vi "SubTest_SelectData.vi"(8 "error in (no error)":errorcluster) -> (0 "error out":errorcluster, 1 "Selected?T":bool)   [LabVIEW 2014, in "TableLogger_CSV_Actor.lvlib" / "TableLogger_CSV_Actor.lvclass"]
uses:
  TableLogger_CSV_Actor.lvclass
  TableLogger_Actor/TableLoggerConfig.ctl
  TableLogger_Actor/TableLoggerTypes.ctl
  TableLogger_Actor/TableLoggerBackupConfig.ctl
  TableLogger_Actor/SelectConditionCriteria.ctl
  TableLogger_SQLite_Actor/SelectConditions.ctl
  TableLogger_Actor/TableLogger_Actor.lvlib
panel:
  # "This example to check CSV update on Tablelogger"
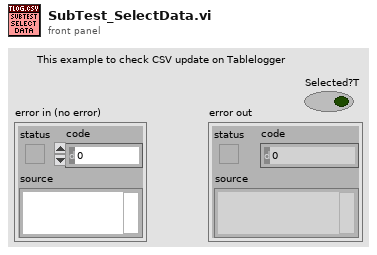
[diagram p1: front panel]
types:
  T1 = typedef "TableLogger_Actor.lvlib/SelectConditionCriteria.ctl" = cluster{"Condition Data":variant[], "Recent N.Rows":string, "Select Type":T2}
  T2 = typedef "TableLogger_Actor.lvlib/SelectConditions.ctl" = enum16{"Select All", "AND Operator", "Recent Rows", "OR Operator", "BETWEEN Operator"}
  T3 = cluster{"Numeric Data":i32, "Float Data":dbl, "String Data":string, "Enum Data":enum16{"Enum Item 1", "Enum Item 2"}, "Array Data 2":i32[], "Cluster 2":cluster{"String":string, "Array Data 2":i32[]}, "Cluster 3":cluster{"Cluster78":cluster{"Array Data 2":i32[]}}, "Enum Data 2":enum16{"Enum Item 1", "Enum Item 2"}, "String Data 2":string, "Float Data 2":dbl, "Array Data":i32[], "Array A":cluster{"String A":string, "Array B":cluster{"String B":string, "Array B 2":cluster{"String B":string}[]}[], "Array B 2":cluster{"String B":string}[]}[]}[]
  T4 = typedef "TableLogger_Actor.lvlib/TableLoggerConfig.ctl" = cluster{"TableLogger":T5, "DB File Path":path, "DB Backup Config":T6}
  T5 = typedef "TableLogger_Actor.lvlib/TableLoggerTypes.ctl" = enum16{"CSV Logger", "SQLite Logger"}
  T6 = typedef "TableLogger_Actor.lvlib/TableLoggerBackupConfig.ctl" = cluster{"Directory":path, "UTC Time Format":bool, "On Launch":bool, "Interval (Hours)":dbl, "Size Multiples (Bytes)":i32}
  T7 = cluster{"Numeric Data":i32, "Float Data":dbl, "String Data":string, "Enum Data":enum16{"Enum Item 1", "Enum Item 2"}}
  T8 = cluster{"Test Start Timestamp":timestamp, "Test End Timestamp":timestamp, "Test Jig Location":string, "Location Time Offset":string, "Test Jig ID":string, "Test Jig Fluid":enum16{"Liquid", "Gas"}, "Test Jig Flow":enum16{"Low", "High"}, "Control Board SN":string, "Site Number":i32, "Operator ID":string, "Operation Number":string, "DUT Serial Number":string, "DUT Product Number":string, "DUT Flow Range":i32, "DUT FW Revision":string, "DUT TP1 Offset":dbl, "DUT TP2 Offset":dbl, "DUT Cut Off1":dbl, "DUT Cut Off2":dbl, "PreCal Flow Meas":cluster{"FC Flow Set":dbl, "FM Flow Measure":dbl, "UUT Data":dbl}[], "PostCal Flow Meas":cluster{"FC Flow Set":dbl, "FM Flow Measure":dbl, "UUT Data":dbl}[], "DUT_Coeff":dbl[], "DUT_Flow_Error":dbl[], "Calibration Result":enum16{"Pass", "Fail"}}
  T9 = cluster{"Numeric Data":i32, "Float Data":dbl, "String Data":string, "Enum Data":enum16{"Enum Item 1", "Enum Item 2"}, "Array Data 2":i32[], "Cluster 2":cluster{"String":string, "Array Data 2":i32[]}, "Cluster 3":cluster{"Cluster78":cluster{"Array Data 2":i32[]}}, "Enum Data 2":enum16{"Enum Item 1", "Enum Item 2"}, "String Data 2":string, "Float Data 2":dbl, "Array Data":i32[], "Array A":cluster{"String A":string, "Array B":cluster{"String B":string, "Array B 2":cluster{"String B":string}[]}[], "Array B 2":cluster{"String B":string}[]}[]}
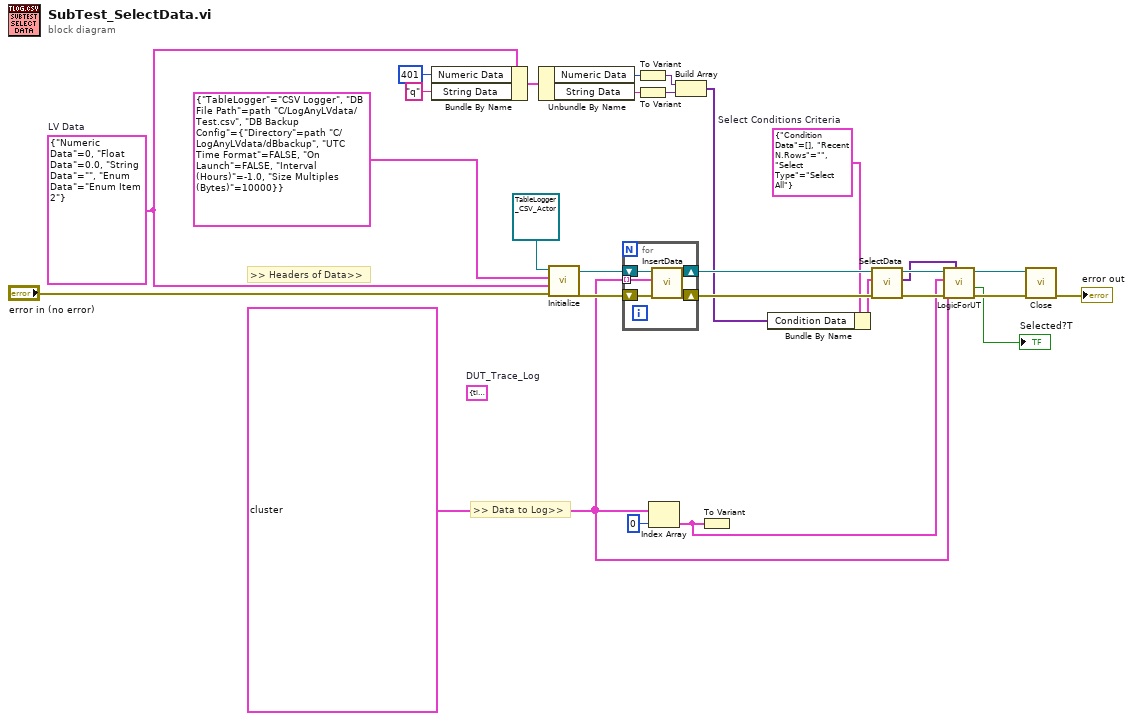
[diagram p0: block diagram]
diagram:
  w3 = T1 {"Condition Data"=[], "Recent N.Rows"="", "Select Type"=enum."Select All"}  # Select Conditions Criteria
  w15 = T3 [{"Numeric Data"=0, "Float Data"=0.0, "String Data"="", "Enum Data"=enum."Enum Item 1", "Array Data 2"=[0, 0, 0], "Cluster 2"={"String"="", "Array Data 2"=[0, 0, 0]}, "Cluster 3"={"Cluster78"={"Array Data 2"=[0, 0, 0]}}, "Enum Data 2"=enum."Enum Item 1", "String Data 2"="", "Float Data 2"=0.0, "Array Data"=[0, 0, 0, 4], "Array A"=[{"String A"="hello", "Array B"=[{"String B"="uq", "Array B 2"=[{"String B"="u"}, {"String B"="c"}, {"String B"="hello"}]}, {"String B"="c", "Array B 2"=[{"String B"="u"}, {"String B"="c"}, {"String B"="hello"}]}, {"String B"="hello", "Array B 2"=[{"String B"="u"}, {"String B"="c"}, {"String B"="hello"}]}], "Array B 2"=[{"String B"="u"}, {"String B"="c"}, {"String B"="hello"}]}, {"String A"="hello", "Array B"=[{"String B"="uP", "Array B 2"=[{"String B"="u"}, {"String B"="c"}, {"String B"="hello"}]}, {"String B"="c", "Array B 2"=[{"String B"="u"}, {"String B"="c"}, {"String B"="hello"}]}, {"String B"="hello", "Array B 2"=[{"String B"="u"}, {"String B"="c"}, {"String B"="hello"}]}], "Array B 2"=[{"String B"="u"}, {"String B"="c"}, {"String B"="hello"}]}]}, {"Numeric Data"=401, "Float Data"=0.0, "String Data"="q", "Enum Data"=enum."Enum Item 1", "Array Data 2"=[0, 0, 0], "Cluster 2"={"String"="", "Array Data 2"=[0, 0, 0]}, "Cluster 3"={"Cluster78"={"Array Data 2"=[0, 0, 0]}}, "Enum Data 2"=enum."Enum Item 1", "String Data 2"="", "Float Data 2"=0.0, "Array Data"=[0, 0, 0, 4], "Array A"=[{"String A"="hello", "Array B"=[{"String B"="uq", "Array B 2"=[{"String B"="u"}, {"String B"="c"}, {"String B"="hello"}]}, {"String B"="c", "Array B 2"=[{"String B"="u"}, {"String B"="c"}, {"String B"="hello"}]}, {"String B"="hello", "Array B 2"=[{"String B"="u"}, {"String B"="c"}, {"String B"="hello"}]}], "Array B 2"=[{"String B"="u"}, {"String B"="c"}, {"String B"="hello"}]}, {"String A"="hello", "Array B"=[{"String B"="uP", "Array B 2"=[{"String B"="u"}, {"String B"="c"}, {"String B"="hello"}]}, {"String B"="c", "Array B 2"=[{"String B"="u"}, {"String B"="c"}, {"String B"="hello"}]}, {"String B"="hello", "Array B 2"=[{"String B"="u"}, {"String B"="c"}, {"String B"="hello"}]}], "Array B 2"=[{"String B"="u"}, {"String B"="c"}, {"String B"="hello"}]}]}, {"Numeric Data"=0, "Float Data"=0.0, "String Data"="", "Enum Data"=enum."Enum Item 1", "Array Data 2"=[0, 0, 0], "Cluster 2"={"String"="", "Array Data 2"=[0, 0, 0]}, "Cluster 3"={"Cluster78"={"Array Data 2"=[0, 0, 0]}}, "Enum Data 2"=enum."Enum Item 1", "String Data 2"="", "Float Data 2"=0.0, "Array Data"=[0, 0, 0, 4], "Array A"=[{"String A"="hello", "Array B"=[{"String B"="uq", "Array B 2"=[{"String B"="u"}, {"String B"="c"}, {"String B"="hello"}]}, {"String B"="c", "Array B 2"=[{"String B"="u"}, {"String B"="c"}, {"String B"="hello"}]}, {"String B"="hello", "Array B 2"=[{"String B"="u"}, {"String B"="c"}, {"String B"="hello"}]}], "Array B 2"=[{"String B"="u"}, {"String B"="c"}, {"String B"="hello"}]}, {"String A"="hello", "Array B"=[{"String B"="uP", "Array B 2"=[{"String B"="u"}, {"String B"="c"}, {"String B"="hello"}]}, {"String B"="c", "Array B 2"=[{"String B"="u"}, {"String B"="c"}, {"String B"="hello"}]}, {"String B"="hello", "Array B 2"=[{"String B"="u"}, {"String B"="c"}, {"String B"="hello"}]}], "Array B 2"=[{"String B"="u"}, {"String B"="c"}, {"String B"="hello"}]}]}, {"Numeric Data"=0, "Float Data"=0.0, "String Data"="", "Enum Data"=enum."Enum Item 1", "Array Data 2"=[0, 0, 0], "Cluster 2"={"String"="", "Array Data 2"=[0, 0, 0]}, "Cluster 3"={"Cluster78"={"Array Data 2"=[0, 0, 0]}}, "Enum Data 2"=enum."Enum Item 1", "String Data 2"="", "Float Data 2"=0.0, "Array Data"=[0, 0, 0, 4], "Array A"=[{"String A"="hello", "Array B"=[{"String B"="uq", "Array B 2"=[{"String B"="u"}, {"String B"="c"}, {"String B"="hello"}]}, {"String B"="c", "Array B 2"=[{"String B"="u"}, {"String B"="c"}, {"String B"="hello"}]}, {"String B"="hello", "Array B 2"=[{"String B"="u"}, {"String B"="c"}, {"String B"="hello"}]}], "Array B 2"=[{"String B"="u"}, {"String B"="c"}, {"String B"="hello"}]}, {"String A"="hello", "Array B"=[{"String B"="uP", "Array B 2"=[{"String B"="u"}, {"String B"="c"}, {"String B"="hello"}]}, {"String B"="c", "Array B 2"=[{"String B"="u"}, {"String B"="c"}, {"String B"="hello"}]}, {"String B"="hello", "Array B 2"=[{"String B"="u"}, {"String B"="c"}, {"String B"="hello"}]}], "Array B 2"=[{"String B"="u"}, {"String B"="c"}, {"String B"="hello"}]}]}, {"Numeric Data"=0, "Float Data"=0.0, "String Data"="", "Enum Data"=enum."Enum Item 1", "Array Data 2"=[0, 0, 0], "Cluster 2"={"String"="", "Array Data 2"=[0, 0, 0]}, "Cluster 3"={"Cluster78"={"Array Data 2"=[0, 0, 0]}}, "Enum Data 2"=enum."Enum Item 1", "String Data 2"="", "Float Data 2"=0.0, "Array Data"=[0, 0, 0, 4], "Array A"=[{"String A"="hello", "Array B"=[{"String B"="uq", "Array B 2"=[{"String B"="u"}, {"String B"="c"}, {"String B"="hello"}]}, {"String B"="c", "Array B 2"=[{"String B"="u"}, {"String B"="c"}, {"String B"="hello"}]}, {"String B"="hello", "Array B 2"=[{"String B"="u"}, {"String B"="c"}, {"String B"="hello"}]}], "Array B 2"=[{"String B"="u"}, {"String B"="c"}, {"String B"="hello"}]}, {"String A"="hello", "Array B"=[{"String B"="uP", "Array B 2"=[{"String B"="u"}, {"String B"="c"}, {"String B"="hello"}]}, {"String B"="c", "Array B 2"=[{"String B"="u"}, {"String B"="c"}, {"String B"="hello"}]}, {"String B"="hello", "Array B 2"=[{"String B"="u"}, {"String B"="c"}, {"String B"="hello"}]}], "Array B 2"=[{"String B"="u"}, {"String B"="c"}, {"String B"="hello"}]}]}, {"Numeric Data"=0, "Float Data"=0.0, "String Data"="", "Enum Data"=enum."Enum Item 1", "Array Data 2"=[0, 0, 0], "Cluster 2"={"String"="", "Array Data 2"=[0, 0, 0]}, "Cluster 3"={"Cluster78"={"Array Data 2"=[0, 0, 0]}}, "Enum Data 2"=enum."Enum Item 1", "String Data 2"="", "Float Data 2"=0.0, "Array Data"=[0, 0, 0, 4], "Array A"=[{"String A"="hello", "Array B"=[{"String B"="uq", "Array B 2"=[{"String B"="u"}, {"String B"="c"}, {"String B"="hello"}]}, {"String B"="c", "Array B 2"=[{"String B"="u"}, {"String B"="c"}, {"String B"="hello"}]}, {"String B"="hello", "Array B 2"=[{"String B"="u"}, {"String B"="c"}, {"String B"="hello"}]}], "Array B 2"=[{"String B"="u"}, {"String B"="c"}, {"String B"="hello"}]}, {"String A"="hello", "Array B"=[{"String B"="uP", "Array B 2"=[{"String B"="u"}, {"String B"="c"}, {"String B"="hello"}]}, {"String B"="c", "Array B 2"=[{"String B"="u"}, {"String B"="c"}, {"String B"="hello"}]}, {"String B"="hello", "Array B 2"=[{"String B"="u"}, {"String B"="c"}, {"String B"="hello"}]}], "Array B 2"=[{"String B"="u"}, {"String B"="c"}, {"String B"="hello"}]}]}, {"Numeric Data"=0, "Float Data"=0.0, "String Data"="", "Enum Data"=enum."Enum Item 1", "Array Data 2"=[0, 0, 0], "Cluster 2"={"String"="", "Array Data 2"=[0, 0, 0]}, "Cluster 3"={"Cluster78"={"Array Data 2"=[0, 0, 0]}}, "Enum Data 2"=enum."Enum Item 1", "String Data 2"="", "Float Data 2"=0.0, "Array Data"=[0, 0, 0, 4], "Array A"=[{"String A"="hello", "Array B"=[{"String B"="uq", "Array B 2"=[{"String B"="u"}, {"String B"="c"}, {"String B"="hello"}]}, {"String B"="c", "Array B 2"=[{"String B"="u"}, {"String B"="c"}, {"String B"="hello"}]}, {"String B"="hello", "Array B 2"=[{"String B"="u"}, {"String B"="c"}, {"String B"="hello"}]}], "Array B 2"=[{"String B"="u"}, {"String B"="c"}, {"String B"="hello"}]}, {"String A"="hello", "Array B"=[{"String B"="uP", "Array B 2"=[{"String B"="u"}, {"String B"="c"}, {"String B"="hello"}]}, {"String B"="c", "Array B 2"=[{"String B"="u"}, {"String B"="c"}, {"String B"="hello"}]}, {"String B"="hello", "Array B 2"=[{"String B"="u"}, {"String B"="c"}, {"String B"="hello"}]}], "Array B 2"=[{"String B"="u"}, {"String B"="c"}, {"String B"="hello"}]}]}, {"Numeric Data"=0, "Float Data"=0.0, "String Data"="", "Enum Data"=enum."Enum Item 1", "Array Data 2"=[0, 0, 0], "Cluster 2"={"String"="", "Array Data 2"=[0, 0, 0]}, "Cluster 3"={"Cluster78"={"Array Data 2"=[0, 0, 0]}}, "Enum Data 2"=enum."Enum Item 1", "String Data 2"="", "Float Data 2"=0.0, "Array Data"=[0, 0, 0, 4], "Array A"=[{"String A"="hello", "Array B"=[{"String B"="uq", "Array B 2"=[{"String B"="u"}, {"String B"="c"}, {"String B"="hello"}]}, {"String B"="c", "Array B 2"=[{"String B"="u"}, {"String B"="c"}, {"String B"="hello"}]}, {"String B"="hello", "Array B 2"=[{"String B"="u"}, {"String B"="c"}, {"String B"="hello"}]}], "Array B 2"=[{"String B"="u"}, {"String B"="c"}, {"String B"="hello"}]}, {"String A"="hello", "Array B"=[{"String B"="uP", "Array B 2"=[{"String B"="u"}, {"String B"="c"}, {"String B"="hello"}]}, {"String B"="c", "Array B 2"=[{"String B"="u"}, {"String B"="c"}, {"String B"="hello"}]}, {"String B"="hello", "Array B 2"=[{"String B"="u"}, {"String B"="c"}, {"String B"="hello"}]}], "Array B 2"=[{"String B"="u"}, {"String B"="c"}, {"String B"="hello"}]}]}, {"Numeric Data"=0, "Float Data"=0.0, "String Data"="", "Enum Data"=enum."Enum Item 1", "Array Data 2"=[0, 0, 0], "Cluster 2"={"String"="", "Array Data 2"=[0, 0, 0]}, "Cluster 3"={"Cluster78"={"Array Data 2"=[0, 0, 0]}}, "Enum Data 2"=enum."Enum Item 1", "String Data 2"="", "Float Data 2"=0.0, "Array Data"=[0, 0, 0, 4], "Array A"=[{"String A"="hello", "Array B"=[{"String B"="uq", "Array B 2"=[{"String B"="u"}, {"String B"="c"}, {"String B"="hello"}]}, {"String B"="c", "Array B 2"=[{"String B"="u"}, {"String B"="c"}, {"String B"="hello"}]}, {"String B"="hello", "Array B 2"=[{"String B"="u"}, {"String B"="c"}, {"String B"="hello"}]}], "Array B 2"=[{"String B"="u"}, {"String B"="c"}, {"String B"="hello"}]}, {"String A"="hello", "Array B"=[{"String B"="uP", "Array B 2"=[{"String B"="u"}, {"String B"="c"}, {"String B"="hello"}]}, {"String B"="c", "Array B 2"=[{"String B"="u"}, {"String B"="c"}, {"String B"="hello"}]}, {"String B"="hello", "Array B 2"=[{"String B"="u"}, {"String B"="c"}, {"String B"="hello"}]}], "Array B 2"=[{"String B"="u"}, {"String B"="c"}, {"String B"="hello"}]}]}, {"Numeric Data"=0, "Float Data"=0.0, "String Data"="", "Enum Data"=enum."Enum Item 1", "Array Data 2"=[0, 0, 0], "Cluster 2"={"String"="", "Array Data 2"=[0, 0, 0]}, "Cluster 3"={"Cluster78"={"Array Data 2"=[0, 0, 0]}}, "Enum Data 2"=enum."Enum Item 1", "String Data 2"="", "Float Data 2"=0.0, "Array Data"=[0, 0, 0, 4], "Array A"=[{"String A"="hello", "Array B"=[{"String B"="uq", "Array B 2"=[{"String B"="u"}, {"String B"="c"}, {"String B"="hello"}]}, {"String B"="c", "Array B 2"=[{"String B"="u"}, {"String B"="c"}, {"String B"="hello"}]}, {"String B"="hello", "Array B 2"=[{"String B"="u"}, {"String B"="c"}, {"String B"="hello"}]}], "Array B 2"=[{"String B"="u"}, {"String B"="c"}, {"String B"="hello"}]}, {"String A"="hello", "Array B"=[{"String B"="uP", "Array B 2"=[{"String B"="u"}, {"String B"="c"}, {"String B"="hello"}]}, {"String B"="c", "Array B 2"=[{"String B"="u"}, {"String B"="c"}, {"String B"="hello"}]}, {"String B"="hello", "Array B 2"=[{"String B"="u"}, {"String B"="c"}, {"String B"="hello"}]}], "Array B 2"=[{"String B"="u"}, {"String B"="c"}, {"String B"="hello"}]}]}, {"Numeric Data"=0, "Float Data"=0.0, "String Data"="", "Enum Data"=enum."Enum Item 1", "Array Data 2"=[0, 0, 0], "Cluster 2"={"String"="", "Array Data 2"=[0, 0, 0]}, "Cluster 3"={"Cluster78"={"Array Data 2"=[0, 0, 0]}}, "Enum Data 2"=enum."Enum Item 1", "String Data 2"="", "Float Data 2"=0.0, "Array Data"=[0, 0, 0, 4], "Array A"=[{"String A"="hello", "Array B"=[{"String B"="uq", "Array B 2"=[{"String B"="u"}, {"String B"="c"}, {"String B"="hello"}]}, {"String B"="c", "Array B 2"=[{"String B"="u"}, {"String B"="c"}, {"String B"="hello"}]}, {"String B"="hello", "Array B 2"=[{"String B"="u"}, {"String B"="c"}, {"String B"="hello"}]}], "Array B 2"=[{"String B"="u"}, {"String B"="c"}, {"String B"="hello"}]}, {"String A"="hello", "Array B"=[{"String B"="uP", "Array B 2"=[{"String B"="u"}, {"String B"="c"}, {"String B"="hello"}]}, {"String B"="c", "Array B 2"=[{"String B"="u"}, {"String B"="c"}, {"String B"="hello"}]}, {"String B"="hello", "Array B 2"=[{"String B"="u"}, {"String B"="c"}, {"String B"="hello"}]}], "Array B 2"=[{"String B"="u"}, {"String B"="c"}, {"String B"="hello"}]}]}, {"Numeric Data"=401, "Float Data"=0.0, "String Data"="q", "Enum Data"=enum."Enum Item 1", "Array Data 2"=[0, 0, 0], "Cluster 2"={"String"="", "Array Data 2"=[0, 0, 0]}, "Cluster 3"={"Cluster78"={"Array Data 2"=[0, 0, 0]}}, "Enum Data 2"=enum."Enum Item 1", "String Data 2"="", "Float Data 2"=0.0, "Array Data"=[0, 0, 0, 4], "Array A"=[{"String A"="hello", "Array B"=[{"String B"="uq", "Array B 2"=[{"String B"="u"}, {"String B"="c"}, {"String B"="hello"}]}, {"String B"="c", "Array B 2"=[{"String B"="u"}, {"String B"="c"}, {"String B"="hello"}]}, {"String B"="hello", "Array B 2"=[{"String B"="u"}, {"String B"="c"}, {"String B"="hello"}]}], "Array B 2"=[{"String B"="u"}, {"String B"="c"}, {"String B"="hello"}]}, {"String A"="hello", "Array B"=[{"String B"="uP", "Array B 2"=[{"String B"="u"}, {"String B"="c"}, {"String B"="hello"}]}, {"String B"="c", "Array B 2"=[{"String B"="u"}, {"String B"="c"}, {"String B"="hello"}]}, {"String B"="hello", "Array B 2"=[{"String B"="u"}, {"String B"="c"}, {"String B"="hello"}]}], "Array B 2"=[{"String B"="u"}, {"String B"="c"}, {"String B"="hello"}]}]}]
  w5 = T7 {"Numeric Data"=0, "Float Data"=0.0, "String Data"="", "Enum Data"=enum."Enum Item 2"}  # LV Data
  (unwired) T8 {"Test Start Timestamp"=timestamp(0 s since 1904-01-01), "Test End Timestamp"=timestamp(0 s since 1904-01-01), "Test Jig Location"="asdf", "Location Time Offset"="wer", "Test Jig ID"="xcv", "Test Jig Fluid"=enum."Gas", "Test Jig Flow"=enum."High", "Control Board SN"="fgh", "Site Number"=23, "Operator ID"="op", "Operation Number"="op", "DUT Serial Number"="dt", "DUT Product Number"="dt", "DUT Flow Range"=23, "DUT FW Revision"="asdf", "DUT TP1 Offset"=24.0, "DUT TP2 Offset"=546.0, "DUT Cut Off1"=34.0, "DUT Cut Off2"=453.0, "PreCal Flow Meas"=[{"FC Flow Set"=1.0, "FM Flow Measure"=0.0, "UUT Data"=0.0}, {"FC Flow Set"=2.0, "FM Flow Measure"=0.0, "UUT Data"=0.0}, {"FC Flow Set"=3.0, "FM Flow Measure"=0.0, "UUT Data"=0.0}], "PostCal Flow Meas"=[{"FC Flow Set"=1.0, "FM Flow Measure"=0.0, "UUT Data"=0.0}, {"FC Flow Set"=2.0, "FM Flow Measure"=0.0, "UUT Data"=0.0}], "DUT_Coeff"=[1.0, 2.0], "DUT_Flow_Error"=[1.0, 2.0], "Calibration Result"=enum."Fail"}  # DUT_Trace_Log
  # ">> Headers of Data>>"
  # ">> Data to Log>>"
  n1 = Bundle By Name(cluster=w5, "Numeric Data"=401, "String Data"="q") -> (w10:T7)
  n2 = Unbundle By Name(w10) -> ("Numeric Data"=w8:i32, "String Data"=w9:string)
  n3 = call-dynamic "Initialize.vi"("error in (no error)"="error in (no error)", "Data Cluster (for Headers)"=w5, "TableLogger Config"=T4 {"TableLogger"=enum."CSV Logger", "DB File Path"=path "C:/LogAnyLVdata/Test.csv", "DB Backup Config"={"Directory"=path "C:/LogAnyLVdata/dBbackup", "UTC Time Format"=FALSE, "On Launch"=FALSE, "Interval (Hours)"=-1.0, "Size Multiples (Bytes)"=10000}}, "object in"=refnum<class "TableLogger_CSV_Actor.lvclass"> refnum) -> ("error out"=w25:errorcluster, "object out"=w26:refnum<class "TableLogger_CSV_Actor.lvclass">)  [unwired: 6 in]
  n4 = for {
    shift-right: [w30] -> w20
    shift-left: w26 -> [w32]
    shift-right: [w29] -> w21
    shift-left: w25 -> [w31]
    tunnel: w15 -> [w28] mode=indexing
    n5 = call-dynamic "InsertData.vi"("error in (no error)"=w31, "Data Cluster"=w28, "object in"=w32) -> ("error out"=w29:errorcluster, "object out"=w30:refnum<class "TableLogger_CSV_Actor.lvclass">)  [unwired: 7 in]
  }
  n6 = To Variant(anything=w8) -> (Variant=w7:variant)
  n7 = To Variant(anything=w9) -> (Variant=w6:variant)
  n8 = Index Array(array=w15, index=0) -> (element=w1:T9)
  n9 = Build Array(w7, w6) -> (w4:variant[])
  n10 = To Variant(anything=w1) -> ()  [unwired: 1 out]
  n11 = Bundle By Name(cluster=w3, "Condition Data"=w4) -> (w2:T1)
  n12 = call-dynamic "SelectData.vi"("error in (no error)"=w21, "Select Conditions Criteria"=w2, "object in"=w20) -> ("error out"=w27:errorcluster, "Data Clusters"=w14:variant[], "object out"=w16:refnum<class "TableLogger_CSV_Actor.lvclass">)  [unwired: 6 in]
  n13 = call "LogicForUT.vi"("Data Clusters"=w14, "error in (no error)"=w27, "Array"=w15, "LV Data"=w1, "TableLogger_CSV_Actor in"=w16) -> ("error out"=w17:errorcluster, "Selected?T"=→"Selected?T":bool)  [unwired: 3 in, 2 out]
  n14 = call-dynamic "Close.vi"("error in (no error)"=w17, "object in"=w16) -> ("error out"=→"error out":errorcluster)  [unwired: 8 in, 1 out]
